vi "Initialize Workspace Control Refs.vi"(9 "State Variables in":T1, 10 "Item.Data":T8, 11 "NIVS.Gateway IP Address":string) -> (0 "error out":errorcluster, 3 "State Variables out":T1)   [LabVIEW 2015, in "Diagnostics Addon Shared.lvlib"]
uses:
  Diagnostics Addon Shared.lvlib
  <vilib>/NI Veristand/Display Template Support/Display Template Support.llb/cluster_Screen Item Settings.ctl
  <vilib>/NI Veristand/Display Template Support/Display Template Support.llb/cluster_Graph Scale Settings.ctl
  <vilib>/NI Veristand/Display Template Support/Display Template Support.llb/cluster_Graph Plot Settings.ctl
  Types/Workspace.State.ctl
  Types/UI.Refs.ctl
  Types/Command.ctl
  <vilib>/NI Veristand/Display Template Support/Display Template Support.llb/enum_Display Template Handler Minimal To Workspace.ctl
  Types/Workspace.SavedState.ctl
  NationalInstruments.VeriStand.SystemStorage
  <vilib>/NI Veristand/Execution/Workspace/WorkspaceAPI.ctl
  NationalInstruments.VeriStand.ClientAPI
  <vilib>/NI Veristand/Display Template Support/Display Template Support.llb/enum_Display Template Handler Minimal To Widget Msg.ctl
  <vilib>/NI Veristand/Execution/Workspace/SystemStateRegEventRef.ctl
  <vilib>/NI Veristand/Execution/Workspace/Target State Info.ctl
  <vilib>/NI Veristand/Execution/Workspace/Target State.ctl
  <vilib>/NI Veristand/Execution/Workspace/SystemStateEventRef.ctl
  Types/Protocol.ctl
  <vilib>/NI Veristand/Execution/Workspace/NI_VS Workspace ExecutionAPI.lvlib
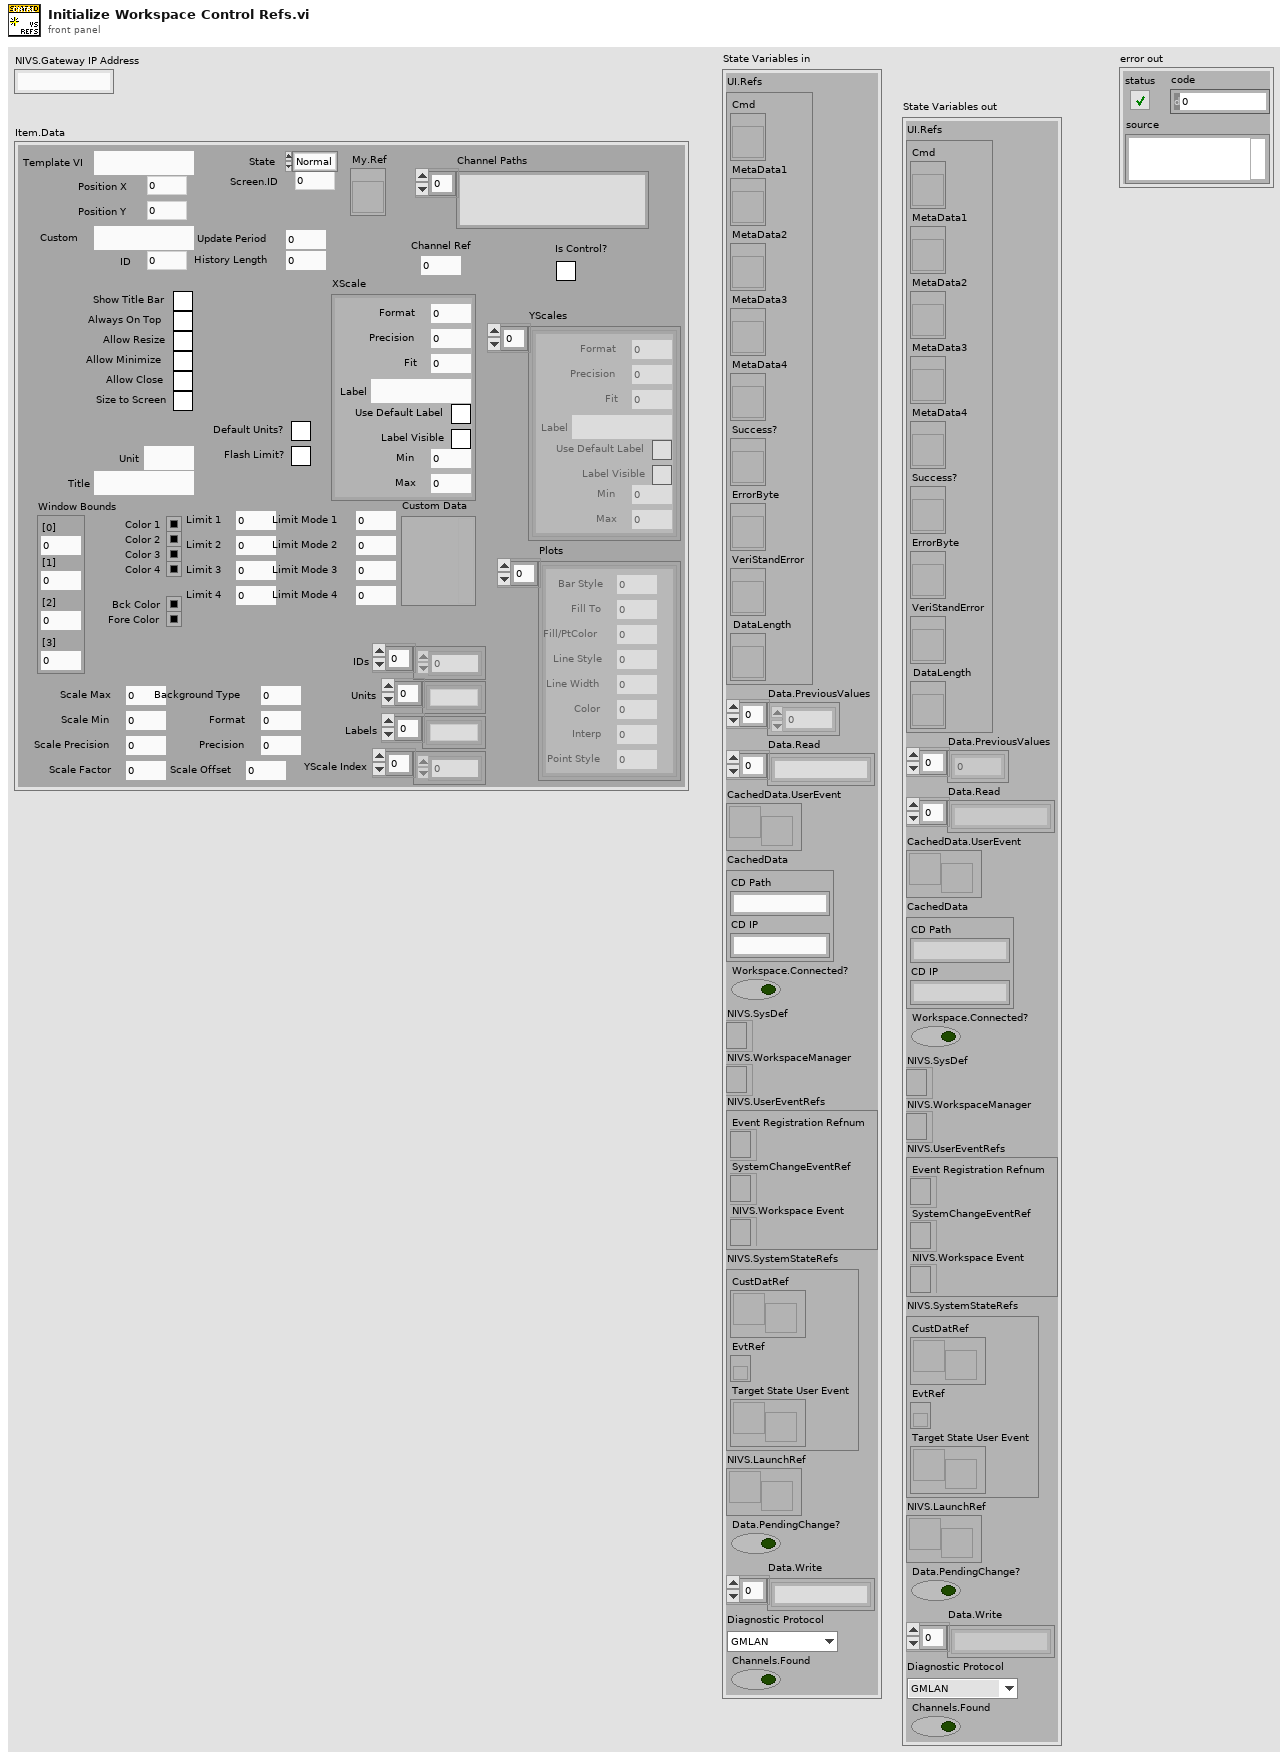
[diagram p1: front panel]
types:
  T1 = typedef "Diagnostics Addon Shared.lvlib/Workspace.State.ctl" = cluster{"UI.Refs":T2, "Data.PreviousValues":dbl[], "Data.Read":string[], "CachedData.UserEvent":refnum<user-event>, "CachedData":T3, "Workspace.Connected?":bool, "NIVS.SysDef":refnum<k24>, "NIVS.WorkspaceManager":T4, "NIVS.UserEventRefs":cluster{"Event Registration Refnum":refnum<event-registration>, "SystemChangeEventRef":T5, "NIVS.Workspace Event":refnum<event-registration>}, "NIVS.SystemStateRefs":T6, "NIVS.LaunchRef":refnum<user-event>, "Data.PendingChange?":bool, "Data.Write":string[], "Diagnostic Protocol":T7, "Channels.Found":bool}
  T2 = typedef "Diagnostics Addon Shared.lvlib/UI.Refs.ctl" = cluster{"Cmd":refnum<vi>, "MetaData1":refnum<vi>, "MetaData2":refnum<vi>, "MetaData3":refnum<vi>, "MetaData4":refnum<vi>, "Success?":refnum<vi>, "ErrorByte":refnum<vi>, "VeriStandError":refnum<vi>, "DataLength":refnum<vi>}
  T3 = typedef "Diagnostics Addon Shared.lvlib/Workspace.SavedState.ctl" = cluster{"CD Path":string, "CD IP":string}
  T4 = typedef "NI_VS Workspace ExecutionAPI.lvlib/WorkspaceAPI.ctl" = refnum<k24>
  T5 = typedef "NI_VS Workspace ExecutionAPI.lvlib/SystemStateRegEventRef.ctl" = refnum<event-registration>
  T6 = typedef "NI_VS Workspace ExecutionAPI.lvlib/SystemStateEventRef.ctl" = cluster{"CustDatRef":refnum<user-event>, "EvtRef":refnum<k27>, "Target State User Event":refnum<user-event>}
  T7 = typedef "Diagnostics Addon Shared.lvlib/Protocol.ctl" = enum16{"GMLAN", "KWP-2000", "UDS"}
  T8 = typedef "cluster_Screen Item Settings.ctl" = cluster{"Template VI":string, "Position X":i32, "Position Y":i32, "Custom":string, "Show Title Bar":bool, "ID":i32, "Always On Top":bool, "Allow Resize":bool, "Allow Minimize":bool, "Allow Close":bool, "Size to Screen":bool, "Screen.ID":i32, "State":enum16{"Normal", "New"}, "Title":string, "Window Bounds":cluster{"[0]":i16, "[1]":i16, "[2]":i16, "[3]":i16}, "Channel Ref":u64, "Unit":string, "Default Units?":bool, "Flash Limit?":bool, "Color 1":u32, "Color 2":u32, "Color 3":u32, "Color 4":u32, "Bck Color":u32, "Fore Color":u32, "Limit 1":dbl, "Limit 2":dbl, "Limit 3":dbl, "Limit 4":dbl, "Limit Mode 1":i32, "Limit Mode 2":i32, "Limit Mode 3":i32, "Limit Mode 4":i32, "Scale Precision":i32, "Scale Min":dbl, "Scale Max":dbl, "Format":i32, "Precision":i32, "Background Type":i32, "IDs":i32[], "Units":string[], "Labels":string[], "Scale Factor":dbl, "Scale Offset":dbl, "YScale Index":u32[], "XScale":T9, "YScales":T9[], "Plots":T10[], "Update Period":dbl, "History Length":dbl, "My.Ref":refnum<vi>, "Is Control?":bool, "Channel Paths":string[], "Custom Data":variant}
  T9 = typedef "cluster_Graph Scale Settings.ctl" = cluster{"Format":u8, "Precision":u8, "Fit":u8, "Label":string, "Use Default Label":bool, "Label Visible":bool, "Min":dbl, "Max":dbl}
  T10 = typedef "cluster_Graph Plot Settings.ctl" = cluster{"Bar Style":u8, "Fill To":i16, "Fill/PtColor":u32, "Line Style":u8, "Line Width":u8, "Color":u32, "Interp":u8, "Point Style":u8}
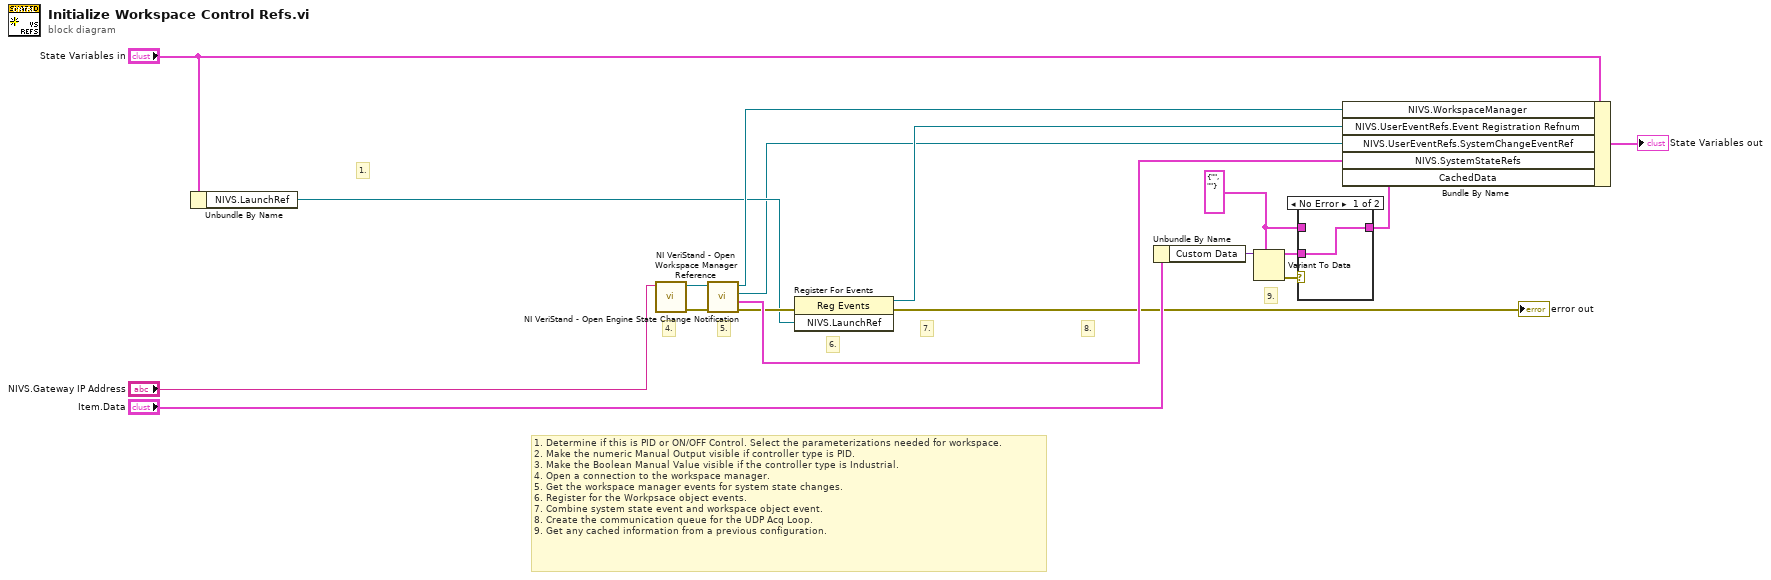
[diagram p0: block diagram]
diagram:
  w4 = T3 {"CD Path"="", "CD IP"=""} ("CachedData")
  # "1. Determine if this is PID or ON/OFF Control. Select the parameterizations needed for workspace.\n2. Make the numeric Manual Output visible if controller type is PID.\n3. Make the Boolean Manual Value visible if the controller type is Industrial.\n4. Open a connection to the workspace manager.\n5. Get the workspace manager events for system state changes.\n6. Register for the Workpsace object events.\n7. Combine system state event and workspace object event.\n8. Create the communication queue for the UDP Acq Loop.\n9. Get any cached information from a previous configuration."
  # "9."
  # "8."
  # "7."
  # "6."
  # "5."
  # "4."
  # "1."
  n1 = Unbundle By Name("State Variables in") -> ("NIVS.LaunchRef"=w6:refnum<user-event>)
  n2 = call <vilib>:"NI VeriStand - Open Workspace Manager Reference.vi"("Gateway IP Address (\"\": localhost)"="NIVS.Gateway IP Address") -> ("error out"=w10:errorcluster, "WorkspaceManager"=w15:T4)  [unwired: 9 in]
  n3 = call <vilib>:"NI VeriStand - Open Engine State Change Notification.vi"("error in (no error)"=w10, "WorkspaceManager in"=w15) -> ("error out"=w7:errorcluster, "SystemStateRefs"=w14:T6, "SystemChangeEventRef"=w1:T5, "WorkspaceManager out"=w8:T4)  [unwired: 6 in]
  n4 = register-events(error in=w7, w6) -> (reference out=w2:refnum<event-registration>, error out=→"error out":errorcluster)  [unwired: 1 in]
  n5 = Unbundle By Name("Item.Data") -> ("Custom Data"=w11:variant)
  n6 = Variant To Data(type=w4, Variant=w11) -> (data=w13:T3, error out=w12:errorcluster)  [unwired: 1 in]
  n7 = case shown="No Error" w12 {
    tunnel: w13 -> [w19 _]
    tunnel: [w19 w20] -> w3
    tunnel: w4 -> [_ w20]
    frame No Error {
    }
    frame Error {
    }
  }
  n8 = Bundle By Name(cluster="State Variables in", "NIVS.WorkspaceManager"=w8, "NIVS.UserEventRefs.Event Registration Refnum"=w2, "NIVS.UserEventRefs.SystemChangeEventRef"=w1, "NIVS.SystemStateRefs"=w14, "CachedData"=w3) -> (→"State Variables out":T1)
